vi "Dashboard Main.vi"() -> ()   [LabVIEW 2015]
uses:
  <vilib>/Utility/miscctls.llb/LVRowAndColumnTypeDef.ctl
  <vilib>/event_ctls.llb/eventvkey.ctl
  <vilib>/Rock Robotics/WPI/Dashboard/WPI_DashboardLogging Global.vi
  <vilib>/Rock Robotics/Network Tables/NT Read Boolean.vi
  <vilib>/Rock Robotics/Network Tables/NT Read Numeric Array.vi
  <vilib>/Utility/config.llb/Write Key (String).vi
  <vilib>/Utility/config.llb/Write Key (I32).vi
  <vilib>/Utility/config.llb/NI_LVConfig.lvlib
panel:
  in  "TCP":refnum<k5>
  in  "Rec Mode":enum32{"Stop", "Record", "Playback"}(radio)
  in  "Vision":u16(ring) items=["Camera Off", "USB Camera SW", "USB Camera HW", "IP Camera"]
  out "Camera IP":string
  out "Image Message":string="Timeout in Camera Communications"
  in  "Dashboard Tab":T1(tab)
  out "Joystick":dbl(knob) scale=0.0..360.0
  out "Encodeur 4":dbl
  out "Encodeur 3":dbl
  out "Encodeur 2":dbl
  out "encodeur 1":dbl
  in  "Select Auto":string(combo)
  out "NT Connection":bool
  in  "Camera Settings":T2={"Frame Rate"=30, "Compression"=30, "Size"=1} {"Frame Rate" scale=1.0..30.0; "Size" items=["640x480", "320x240", "160x120"]}
  out "MotorChart R":cluster{"Numeric":dbl, "Numeric":dbl}(graph)
  out "MotorChart L":T3(graph)
  out "MotorSliders R":cluster{"MotorSlide1":dbl, "MotorSlide2":dbl} {"MotorSlide2" scale=-1.0..1.0 scale format="%#_2e"; "MotorSlide1" scale=-1.0..1.0 scale format="%#_2e"}
  out "MotorSliders L":T4 {"MotorSlide4 2" scale=0.0..14.0 scale format="%#_2e"; "MotorSlide2" scale=-1.0..1.0 scale format="%#_2e"; "MotorSlide1" scale=-1.0..1.0 scale format="%#_2e"}
  out "orientation swerves":dbl(knob) scale=0.0..360.0
  out "JS1 Z":dbl(slide) scale=-1.0..1.0 scale format="%#_2e"
  out "JS1 Graph":cluster{"X":dbl, "Y":dbl}[](graph)
  out "JS1 Buttons":T5
  out "JS2 Z":dbl(slide) scale=-1.0..1.0 scale format="%#_2e"
  out "JS2 Graph":cluster{"X":dbl, "Y":dbl}[](graph)
  out "JS2 Buttons":T5
  out "Mode":T6(ring)=enum."Auto Disabled"
  in  "DB Camera Config":bool
  out "fps":dbl format="%#.1g"
  out "Mbps":dbl format="%#.1g"
  out "Mbps LED":bool
  in  "DB/String 9":string
  in  "DB/String 8":string
  in  "DB/String 7":string
  in  "DB/String 6":string
  in  "DB/String 5":string
  in  "DB/String 4":string
  in  "DB/String 3":string
  in  "DB/String 2":string
  in  "DB/String 1":string
  in  "DB/String 0":string
  in  "DB/Slider 0":dbl(slide) scale=0.0..5.0
  in  "DB/Slider 1":dbl(slide) scale=0.0..5.0
  in  "DB/Slider 2":dbl(slide) scale=0.0..5.0
  in  "DB/Slider 3":dbl(slide) scale=0.0..5.0
  out "DB/LED 3":bool
  out "DB/LED 2":bool
  out "DB/LED 1":bool
  out "DB/LED 0":bool
  in  "DB/Button 3":bool
  in  "DB/Button 2":bool
  in  "DB/Button 1":bool
  in  "DB/Button 0":bool caption="New Name"
  in  "Test Slider":dbl(slide) scale=0.0..100.0 scale format="%#_3g"
  in  "On/Off":bool caption="Solenoid"
  in  "Test Name":u16(ring) items=["Select the test to run..."]
  in  "Test Tree":string(tree)
  in  "Motor":cluster{"Value":dbl, "Enable":bool} {"Value" scale=-1.0..1.0 scale format="%#_3g"}
  out "Progress":T7 {"Test Progress" scale=0.0..100.0}
  in  "Rev/Fwd":cluster{"Forward":bool, "Reverse":bool}
  in  "Test Ring":u16(ring) items=["Monochrome", "Color"]
  out "Cmd Status":string
  in  "Execute Command":bool
  in  "Command Params":string[][](table)
  in  "Command Selection":i32(listbox)
  in  "CheckList":i32(listbox)
  out "Tree":string(tree)
  out "Camera Image":T8(plugin-control)
  out "Background":bool
  # "Left"
  # "Front"
  # "Right"
  # "Battery"
  # "This tab is a great place for autonomous settings and robot-specific values.\nPlace controls and indicators inside this tab and match name to\nDashboard Variables on robot. You can also delete this comment."
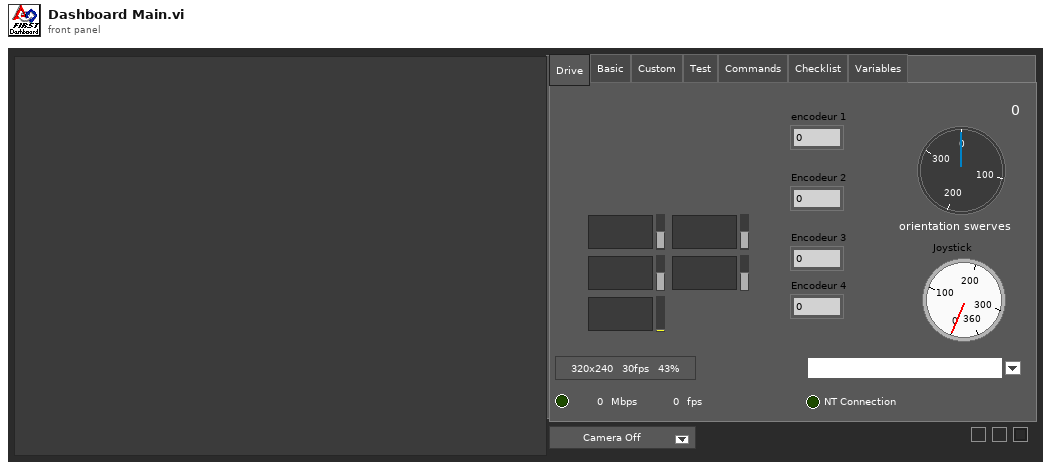
[diagram p1: front panel]
types:
  T1 = enum32{"Drive", "Basic", "Custom", "Test", "Commands", "Checklist", "Variables"}
  T2 = cluster{"Frame Rate":i32, "Compression":i32, "Size":u16}
  T3 = cluster{"Numeric":dbl, "Numeric":dbl, "Battery V":dbl}
  T4 = cluster{"MotorSlide1":dbl, "MotorSlide2":dbl, "MotorSlide4 2":dbl}
  T5 = cluster{bool, bool, bool, bool, bool, bool, bool, bool, bool, bool, bool, bool}
  T6 = enum8{"Tele-Op Disabled", "Tele-Op Enabled", "Auto Disabled", "Auto Enabled", "Test Disabled", "Test Enabled", "Disconnected", "No Code", "E-Stop"}
  T7 = cluster{"Test Progress":u8, "Test Progress Text":string}
  T8 = typedef "IMAQ Image.ctl" = refnum<image>
  T9 = cluster{"IDs":cluster{"RPC field ID":u16, "Unique ID":u16}, "String":string}
  T10 = enum32{"Drive", "Basic", "Custom", "Test", "Checklist", "Variables"}
  T11 = typedef "Image Type" = u32
  T12 = cluster{"Camera Image":refnum<vi>, "Dashboard Tab":refnum<vi>, "Background":refnum<vi>, "Vision":refnum<vi>, "Rec Mode":refnum<vi>, "Test Slider":refnum<vi>, "On/Off ":refnum<vi>, "Test Ring":refnum<vi>, "Rev/Fwd":refnum<vi>, "Test Name":refnum<vi>, "Motor":refnum<vi>, "Progress":refnum<vi>, "CheckList":refnum<vi>, "Tree":refnum<vi>, "Test Tree":refnum<vi>, "Command Params":refnum<vi>, "Command Selection":refnum<vi>, "Execute Command":refnum<vi>, "Cmd Status":refnum<vi>}
  T13 = cluster{"Error Strings":string, "Disable Counts":cluster{u16, u16}, "Rail Faults":cluster{u16, u16, u16}, "Robot IP":string, "DB Mode":u8, "Event Info":cluster{"Name":string, "Type":u8, "Number":u16, "Replay":u8}, "Camera Addr":string}
  T14 = cluster{"Storage":cluster{"Disk Free":u64, "RAM Block":u32, "RAM free":u32}, "CPU Utilization":cluster{"CPU % ISR":sgl, "CPU % Time Crit":sgl, "CPU % Timed Str":sgl, "CPU % High":sgl, "CPU % Above":sgl, "CPU % Normal":sgl, "CPU % Low":sgl}, "CAN":cluster{"% Bus Utilization":sgl, "Bus Off Cnt":u32, "TX_FIFO Full Cnt":u32, "Receive Error Cnt":u8, "Transmit Error Cnt":u8}, "HID":cluster{"HID Outputs":u32, "Rumble Low":u16, "Rumble High":u16}[]}
  T15 = cluster{"Status bits":cluster{"Test Mode":bool, "Autonomous":bool, "Enabled":bool, "Code Start":bool, "Brownout":bool, "Reserved 2":bool, "Reserved 3":bool, "E-Stop":bool}, "Code Trace":cluster{"Disabled":bool, "TeleOp":bool, "Auto":bool, "Test":bool}, "Controller Type":enum16{"unknown", "cRIO", "roboRio"}, "Code?":enum16{"unknown", "noCode", "code"}, "Battery V":dbl}
  T16 = cluster{"Control Bits":cluster{"TestMode":bool, "Autonomous":bool, "Enabled":bool, "FMS Present":bool, bool, bool, bool, "E-Stop":bool}, "Team Station ":u8, "Countdown":sgl, "Joystick Values":cluster{"Axes":dbl[], "Buttons":bool[], "POVs":i16[]}[]}
  T17 = cluster{"Axes":dbl[], "Buttons":bool[], "POVs":i16[]}[]
  T18 = cluster{"Axes":dbl[], "Buttons":bool[], "POVs":i16[]}
  T19 = cluster{"Buttons[0]":bool, "Buttons[1]":bool, "Buttons[2]":bool, "Buttons[3]":bool, "Buttons[4]":bool, "Buttons[5]":bool, "Buttons[6]":bool, "Buttons[7]":bool, "Buttons[8]":bool, "Buttons[9]":bool, "Buttons[10]":bool, "Buttons[11]":bool}
  T20 = typedef "NI_LVConfig.lvlib/Config Data RefNum.ctl" = refnum<k1>
  T21 = cluster{"Operation":enum16{"Update", "Clear"}, "Color Box":u32}[]
  T22 = typedef "eventvkey.ctl" = enum16{"ASCII", "Enter", "Return", "Shift", "Ctrl", "Alt", "Cmd", "Opt", "Caps", "NumLock", "Clear", "Break", "Up", "Down", "Left", "Right", "Insert", "Delete", "Home", "End", "PageUp", "PageDown", "Escape", "Help", "Pause", "ScrollLock", "F1", "F2", "F3", "F4", "F5", "F6", "F7", "F8", "F9", "F10", "F11", "F12", "F13", "F14", "F15", "F16", "F17", "F18", "F19", "F20", "F21", "F22", "F23", "F24", "Play", "VolumeUp", "VolumeDown", "Mute", "Two Byte Char"}
  T23 = cluster{"Image Size":bool, "Image Type":bool, "Pixel Value":bool, "ROI Information":bool, "Zoom Factor":bool}
  T24 = enum8{"Enabled", "Disabled", "Disabled and Grayed Out"}
  T25 = cluster{"Operation":enum16{"Update", "Clear"}, "Color Box":u32}
  T26 = typedef "LVRowAndColumnTypeDef.ctl" = cluster{"Row":i32, "Column":i32}
  T27 = cluster{"Shift":bool, "Ctrl":bool, "Alt":bool, "Cmd":bool, "Opt":bool}
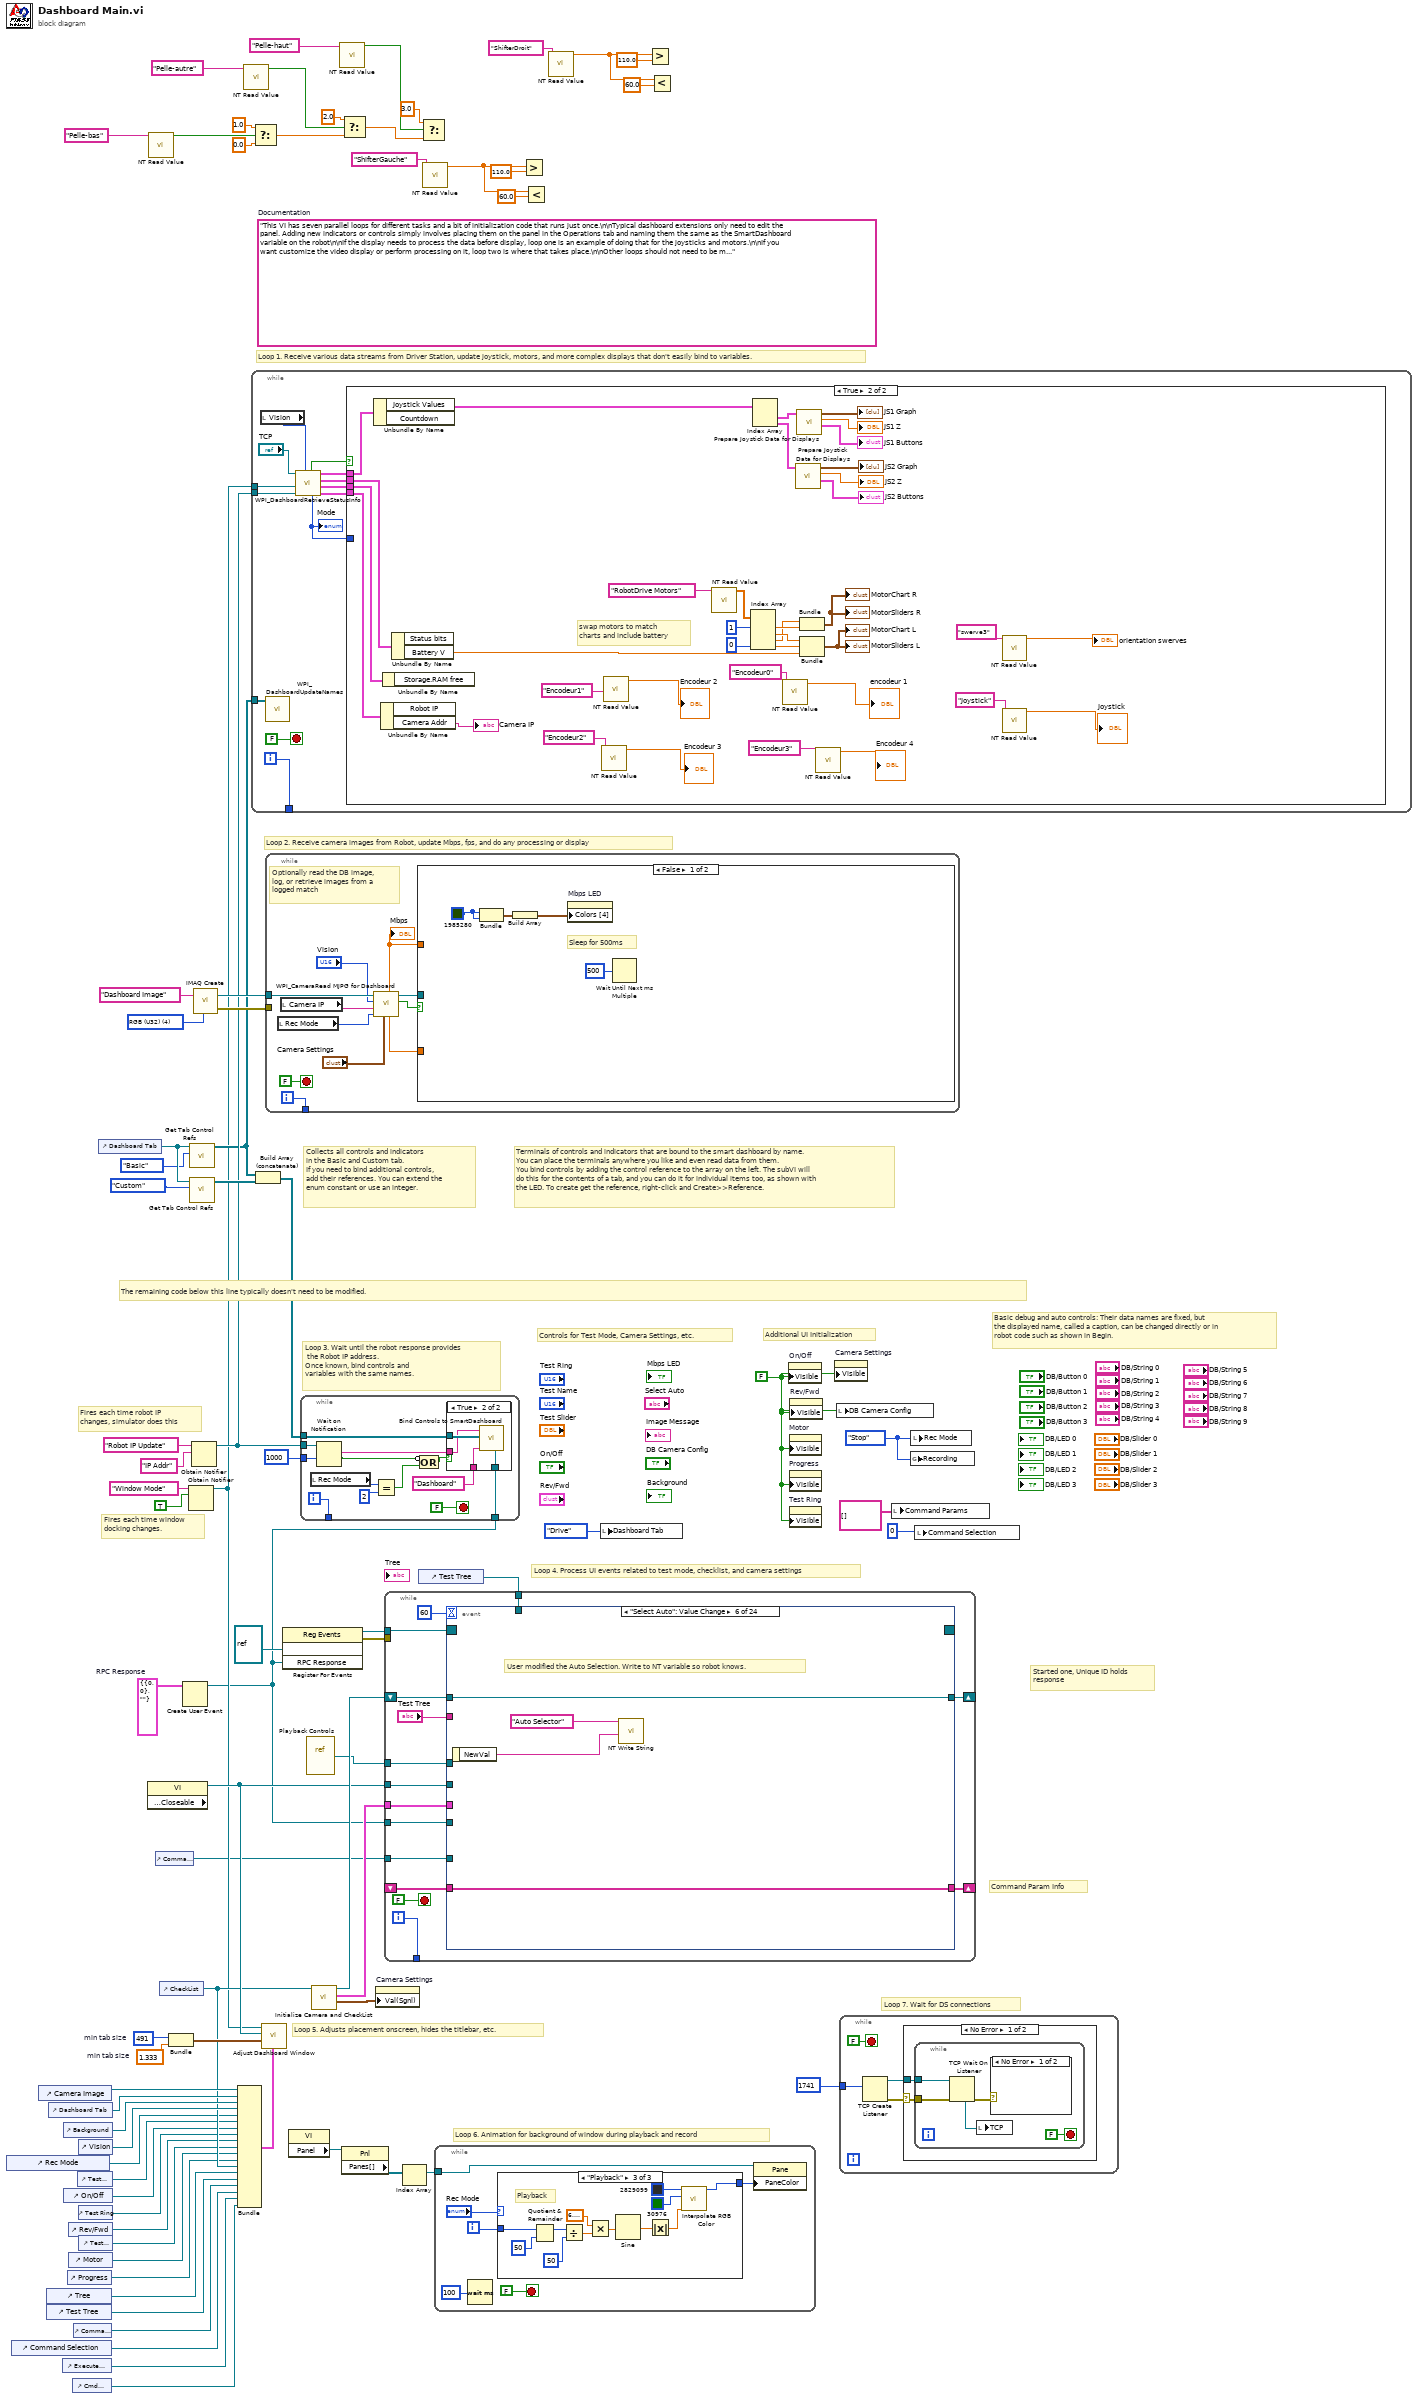
[diagram p0: block diagram]
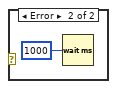
[diagram p2: hidden frame]
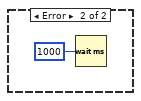
[diagram p3: hidden frame]
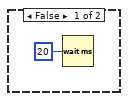
[diagram p4: hidden frame]
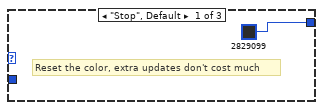
[diagram p5: hidden frame]
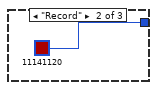
[diagram p6: hidden frame]
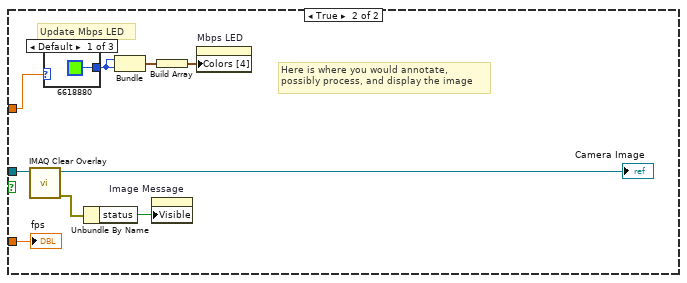
[diagram p8: hidden frame]
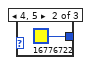
[diagram p9: hidden frame]
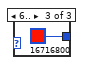
[diagram p10: hidden frame]
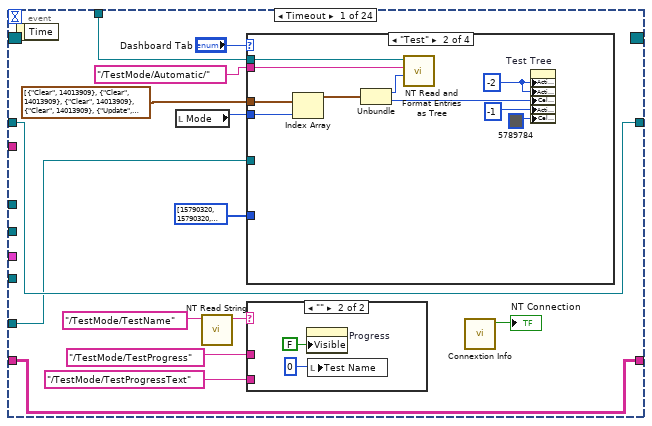
[diagram p11: hidden frame]
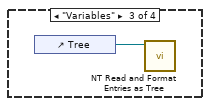
[diagram p13: hidden frame]
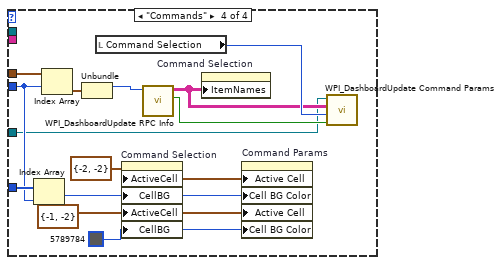
[diagram p14: hidden frame]
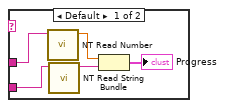
[diagram p15: hidden frame]
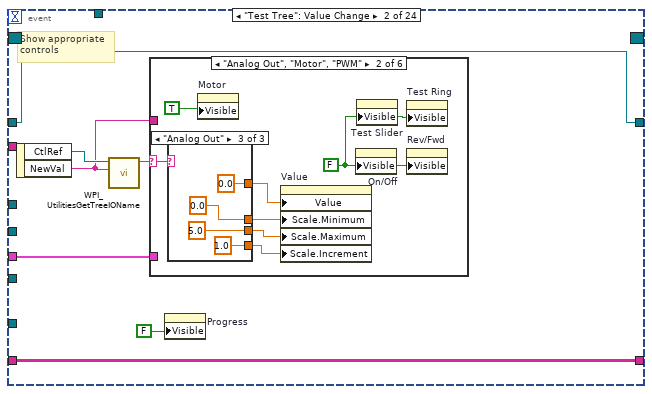
[diagram p16: hidden frame]
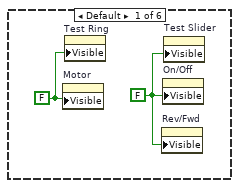
[diagram p17: hidden frame]
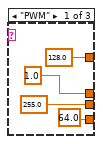
[diagram p18: hidden frame]
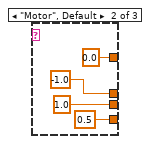
[diagram p19: hidden frame]
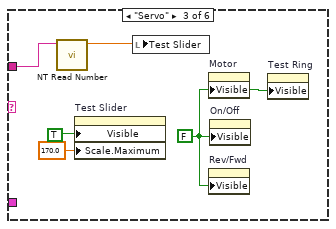
[diagram p20: hidden frame]
diagram:
  w27 = T9 {"IDs"={"RPC field ID"=0, "Unique ID"=0}, "String"=""}  # RPC Response
  w53 = 491  # min tab size
  w52 = 1.333  # min tab size
  w61 = enum32{"Stop", "Record", "Playback"}."Stop" ("Rec Mode")
  w35 = FALSE ("Visible")
  (unwired) "This VI has seven parallel loops for different tasks and a bit of initialization code that runs just once.\n\nTypical dashboard extensions only need to edit the panel. Adding new indicators or controls simply involves placing them on the panel in the Operations tab and naming them the same as the SmartDashboard variable on the robot\n\nIf the display needs to process the data before display, loop one is an example of doing that for the joysticks and motors.\n\nIf you want customize the video display or perform processing on it, loop two is where that takes place.\n\nOther loops should not need to be modified. They are pretty standard, and document the task they perform."  # Documentation
  w81 = T11 4 items=["Grayscale (U8)", "Grayscale (I16)", "Grayscale (SGL)", "Complex (CSG)", "RGB (U32)", "HSL (U32)", "RGB (U64)"] ("Image Type")
  # "Command Param Info"
  # "Started one, Unique ID holds\nresponse"
  # "Loop 7. Wait for DS connections"
  # "Basic debug and auto controls: Their data names are fixed, but\nthe displayed name, called a caption, can be changed directly or in\nrobot code such as shown in Begin."
  # "Controls for Test Mode, Camera Settings, etc."
  # "Additional UI Initialization"
  # "Loop 6. Animation for background of window during playback and record"
  # "Fires each time robot IP\nchanges, simulator does this"
  # "Fires each time window\ndocking changes."
  # "Collects all controls and indicators\nin the Basic and Custom tab.\nIf you need to bind additional controls,\nadd their references. You can extend the\nenum constant or use an integer."
  # "The remaining code below this line typically doesn't need to be modified."
  # "Loop 4. Process UI events related to test mode, checklist, and camera settings"
  # "Terminals of controls and indicators that are bound to the smart dashboard by name.\nYou can place the terminals anywhere you like and even read data from them.\nYou bind controls by adding the control reference to the array on the left. The subVI will\ndo this for the contents of a tab, and you can do it for individual items too, as shown with\nthe LED. To create get the reference, right-click and Create>>Reference."
  # "Loop 3. Wait until the robot response provides\n the Robot IP address.\nOnce known, bind controls and\nvariables with the same names."
  # "Loop 5. Adjusts placement onscreen, hides the titlebar, etc."
  # "Loop 1. Receive various data streams from Driver Station, update joystick, motors, and more complex displays that don't easily bind to variables."
  # "Loop 2. Receive camera images from Robot, update Mbps, fps, and do any processing or display"
  n1 = control-ref of="Rec Mode"() -> (w41:refnum<vi>)
  n2 = control-ref of="Command Selection"() -> (w26:refnum<vi>)
  n3 = control-ref of="Camera Image"() -> (w56:refnum<vi>)
  n4 = control-ref of="Tree"() -> (w45:refnum<vi>)
  n5 = control-ref of="Test Tree"() -> (w44:refnum<vi>)
  n6 = control-ref of="Dashboard Tab"() -> (w55:refnum<vi>)
  n7 = control-ref of="Execute Command"() -> (w28:refnum<vi>)
  n8 = control-ref of="Background"() -> (w50:refnum<vi>)
  n9 = control-ref of="On/Off"() -> (w39:refnum<vi>)
  n10 = control-ref of="Progress"() -> (w36:refnum<vi>)
  n11 = control-ref of="Rev/Fwd"() -> (w37:refnum<vi>)
  n12 = control-ref of="Motor"() -> (w42:refnum<vi>)
  n13 = control-ref of="Cmd Status"() -> (w22:refnum<vi>)
  n14 = control-ref of="Command Params"() -> (w29:refnum<vi>)
  n15 = control-ref of="Test Slider"() -> (w40:refnum<vi>)
  n16 = control-ref of="Vision"() -> (w54:refnum<vi>)
  n17 = control-ref of="Test Ring"() -> (w38:refnum<vi>)
  n18 = control-ref of="Test Name"() -> (w43:refnum<vi>)
  n19 = control-ref of="Dashboard Tab"() -> (w59:refnum<vi>)
  n20 = property class="VI" props=["Front Panel.Closeable"]() -> (reference out=w60:refnum<vi>)  [unwired: 2 in, 2 out]
  n21 = call-poly <vilib>:"NT Read Value.vi"("Name"="Pelle-bas") -> ("Boolean"=w14:bool)  [unwired: 9 in, 1 out]
  n22 = control-ref of="Command Params"() -> (w21:refnum<vi>)
  n23 = control-ref of="CheckList"() -> (w46:refnum<vi>)
  n24 = Bundle("min tab size"=w53, "min tab size"=w52) -> (w51:cluster{"min tab size":i32, "min tab size":dbl})  [unwired: 1 in]
  n25 = Create User Event(user event datatype=w27) -> (user event=w23:refnum<user-event>)  [unwired: 1 in, 1 out]
  n26 = Obtain Notifier(name (unnamed)="Window Mode", notification data type=TRUE) -> (notifier out=w32:refnum<notifier>)  [unwired: 2 in, 2 out]
  n27 = call <vilib>:"Get Tab Control Refs.vi"("Page Index"=T10."Basic" ("Dashboard Tab"), "TabControl in"=w59) -> ("ControlsOnPage"=w33:refnum<vi>[])  [unwired: 9 in]
  n28 = call <vilib>:"Get Tab Control Refs.vi"("Page Index"=T10."Custom" ("Dashboard Tab"), "TabControl in"=w59) -> ("ControlsOnPage"=w58:refnum<vi>[])  [unwired: 9 in]
  n29 = Obtain Notifier(name (unnamed)="Robot IP Update", notification data type="IP Addr" ("name (unnamed)")) -> (notifier out=w34:refnum<notifier>)  [unwired: 2 in, 2 out]
  n30 = call "IMAQ Create"("Image Name"="Dashboard Image", "Image Type"=w81) -> ("New Image"=w79:T8, "error out"=w78:errorcluster)  [unwired: 2 in, 1 out]
  n31 = Bundle("Camera Image"=w56, "Dashboard Tab"=w55, "Background"=w50, "Vision"=w54, "Rec Mode"=w41, "Test Slider"=w40, "On/Off"=w39, "Test Ring"=w38, "Rev/Fwd"=w37, "Test Name"=w43, "Motor"=w42, "Progress"=w36, "CheckList"=w46, "Tree"=w45, "Test Tree"=w44, "Command Params"=w29, "Command Selection"=w26, "Execute Command"=w28, "Cmd Status"=w22) -> (w47:T12)  [unwired: 1 in]
  n32 = call-poly <vilib>:"NT Read Value.vi"("Name"="Pelle-autre") -> ("Boolean"=w12:bool)  [unwired: 9 in, 1 out]
  n33 = while {
    tunnel: [w93] -> _
    tunnel: w34 -> [w87]
    tunnel: w33 -> [w86]
    tunnel: w32 -> [w82]
    i -> [w93]
    stop <- FALSE stop-if-true
    n34 = local read "Vision"() -> (w84:u16)
    n35 = call <vilib>:"WPI_DashboardUpdateNames.vi"("Controls on Tab"=w86) -> ()  [unwired: 11 in]
    n36 = call <vilib>:"WPI_DashboardRetrieveStatusInfo.vi"("Vision"=w84, "Binding Refnum"=w87, "Window Mode Notifier"=w82, "TCP Cnx"="TCP") -> ("Power and Errors"=w88:T13, "Robot Metrics"=w91:T14, "Status Info"=w92:T15, "Control Info"=w89:T16, "Robot Mode"=w85:T6, "Process?"=w90:bool)  [unwired: 2 in]
    "Mode" <- w85
    n37 = case shown="True" w90 {
      tunnel: w92 -> [_ w132]
      tunnel: w91 -> [_ w131]
      tunnel: w89 -> [_ w130]
      tunnel: w88 -> [_ w129]
      tunnel: w85 -> [_ _]
      frame False {
        n38 = Wait (ms)(milliseconds to wait=u32 20) -> ()  [unwired: 1 out]
      }
      frame True {
        # "swap motors to match\ncharts and include battery"
        n39 = Unbundle By Name(w130) -> ("Joystick Values"=w119:T17)  [unwired: 1 out]
        n40 = Unbundle By Name(w129) -> ("Camera Addr"=→"Camera IP":string)  [unwired: 1 out]
        n41 = Unbundle By Name(w131) -> ()  [unwired: 1 out]
        n42 = Unbundle By Name(w132) -> ("Battery V"=w120:dbl)  [unwired: 1 out]
        n43 = call-poly <vilib>:"NT Read Value.vi"("Name"="Encodeur2") -> ("Numeric"=→"Encodeur 3":dbl)  [unwired: 9 in, 1 out]
        n44 = call-poly <vilib>:"NT Read Value.vi"("Name"="Encodeur1") -> ("Numeric"=→"Encodeur 2":dbl)  [unwired: 9 in, 1 out]
        n45 = call-poly <vilib>:"NT Read Value.vi"("Name"="RobotDrive Motors") -> ("Numeric Array"=w108:dbl[])  [unwired: 9 in, 1 out]
        n46 = Index Array(array=w108, index #1=1, index #4=0) -> (element #1=w124:dbl, element #2=w125:dbl, element #3=w123:dbl, element #4=w128:dbl)  [unwired: 2 in]
        n47 = Index Array(array=w119) -> (element #1=w118:T18, element #2=w113:T18)  [unwired: 2 in]
        n48 = call-poly <vilib>:"NT Read Value.vi"("Name"="Encodeur0") -> ("Numeric"=→"encodeur 1":dbl)  [unwired: 9 in, 1 out]
        n49 = call "Prepare Joystick Data for Displays.vi"("Joystick Values"=w113) -> ("Buttons"=→"JS2 Buttons":T19, "Z Axis"=→"JS2 Z":dbl, "Cartesian Data"=→"JS2 Graph":cluster{"X axis":dbl, "X axis":dbl}[])  [unwired: 8 in]
        n50 = call "Prepare Joystick Data for Displays.vi"("Joystick Values"=w118) -> ("Buttons"=→"JS1 Buttons":T19, "Z Axis"=→"JS1 Z":dbl, "Cartesian Data"=→"JS1 Graph":cluster{"X axis":dbl, "X axis":dbl}[])  [unwired: 8 in]
        n51 = Bundle("Numeric"=w123, "Numeric"=w124) -> (→"MotorChart R" →"MotorSliders R":cluster{"Numeric":dbl, "Numeric":dbl})  [unwired: 1 in]
        n52 = Bundle("Numeric"=w125, "Numeric"=w128, "Battery V"=w120) -> (→"MotorChart L" →"MotorSliders L":T3)  [unwired: 1 in]
        n53 = call-poly <vilib>:"NT Read Value.vi"("Name"="Encodeur3") -> ("Numeric"=→"Encodeur 4":dbl)  [unwired: 9 in, 1 out]
        n54 = call-poly <vilib>:"NT Read Value.vi"("Name"="swerve3") -> ("Numeric"=→"orientation swerves":dbl)  [unwired: 9 in, 1 out]
        n55 = call-poly <vilib>:"NT Read Value.vi"("Name"="Joystick") -> ("Numeric"=→"Joystick":dbl)  [unwired: 9 in, 1 out]
      }
    }
  }
  n56 = Select(t=1.0, s=w14, f=0.0) -> (s? t:f=w11:dbl)
  n57 = Build Array (concatenate)(w33, w58) -> (w57:refnum<vi>[])
  n58 = call "Adjust Dashboard Window.vi"("Sizing Refnums"=w47, "Size Constraints"=w51, "VI"=w60, "WIn Mode"=w32) -> ()  [unwired: 8 in]
  n59 = while {
    tunnel: w79 -> [w141]
    tunnel: w78 -> [_]
    tunnel: [w142] -> _
    i -> [w142]
    stop <- FALSE stop-if-true
    # "Optionally read the DB image,\nlog, or retrieve images from a\nlogged match"
    n60 = local read "Rec Mode"() -> (w136:enum32{"Stop", "Record", "Playback"})
    n61 = local read "Camera IP"() -> (w134:string)
    n62 = call <vilib>:"WPI_CameraRead MJPG for Dashboard.vi"("Camera Settings"="Camera Settings", "Rec Mode"=w136, "Camera IP"=w134, "Camera Mode"="Vision", "Refnum in"=w141) -> ("Active"=w139:bool, "Refnum out"=w140:T8, "FPS"=w138:dbl, "Bandwidth (Mbps)"=w133:dbl)  [unwired: 3 in]
    "Mbps" <- w133
    n63 = case shown="False" w139 {
      tunnel: w140 -> [_ w151]
      tunnel: w133 -> [_ w150]
      tunnel: w138 -> [_ w148]
      frame False {
        w144 = u32 1985280 ("Color Box")
        # "Sleep for 500ms"
        n64 = Bundle("Color Box"=w144, "Color Box"=w144) -> (w146:cluster{"Color Box":u32, "Color Box":u32})  [unwired: 1 out]
        n65 = Build Array(w146) -> (w145:cluster{"Color Box":u32, "Color Box":u32}[])
        n66 = property on="Mbps LED" class="Bool (strict)"("Colors [4]"=w145) -> ()  [unwired: 2 in, 2 out]
        n67 = Wait Until Next ms Multiple(millisecond multiple=u32 500) -> ()  [unwired: 1 out]
      }
      frame True {
        # "Here is where you would annotate,\npossibly process, and display the image"
        # "Update Mbps LED"
        n68 = call "IMAQ Clear Overlay"("Image"=w151) -> ("error out"=w155:errorcluster, "Image Out"=→"Camera Image":T8)  [unwired: 2 in, 7 out]
        n69 = case shown="Default" w150 {
          tunnel: [u32 6618880 ("Color Box") u32 16776722 ("Color Box") u32 16716800 ("Color Box")] -> w152
          frame Default {
          }
          frame 4, 5 {
          }
          frame 6.. {
          }
        }
        n70 = Unbundle By Name(w155) -> ("status"=w156:bool)
        n71 = Bundle("Color Box"=w152, "Color Box"=w152) -> (w154:cluster{"Color Box":u32, "Color Box":u32})  [unwired: 1 out]
        n72 = property on="Image Message" class="Str"("Visible"=w156) -> ()  [unwired: 2 in, 2 out]
        n73 = Build Array(w154) -> (w153:cluster{"Color Box":u32, "Color Box":u32}[])
        n74 = property on="Mbps LED" class="Bool (strict)"("Colors [4]"=w153) -> ()  [unwired: 2 in, 2 out]
        "fps" <- w148
      }
    }
  }
  n75 = register-events(refnum<vi> refnum, w23) -> (reference out=w65:refnum<event-registration>, error out=w64:errorcluster)  [unwired: 2 in]
  n76 = property class="VI"() -> ("Panel"=w68:refnum<vi>)  [unwired: 2 in, 2 out]
  n77 = while {
    tunnel: w57 -> [w172]
    tunnel: w34 -> [w170]
    tunnel: [w168] -> _
    tunnel: u32 1000 ("milliseconds to wait") -> [w167]
    tunnel: w23 -> [w160]
    i -> [w168]
    stop <- FALSE stop-if-true
    n78 = local read "Rec Mode"() -> (w163:enum32{"Stop", "Record", "Playback"})
    n79 = Wait on Notification(notifier=w170, timeout in ms (-1)=w167) -> (notification=w169:string, timed out?=w165:bool)  [unwired: 2 in, 2 out]
    n80 = Equal?(x=w163, y=u16 2 ("Rec Mode")) -> (x = y?=w164:bool)
    n81 = Compound Arithmetic op=OR(invert w165, w164) -> (w166:bool)
    n82 = case shown="True" w166 {
      tunnel: w172 -> [_ w176]
      tunnel: w169 -> [_ w175]
      tunnel: "Dashboard" -> [_ w174]
      tunnel: w160 -> [_ w173]
      frame False {
      }
      frame True {
        n83 = call <vilib>:"Bind Controls to SmartDashboard.vi"("RPC ref"=w173, "Client Name"=w174, "Bound Control Refs"=w176, "Server IP Address"=w175) -> ()  [unwired: 8 in]
      }
    }
  }
  n84 = vi-ref "Playback Controls.vi"() -> (w66:refnum<vi>)
  n85 = call "Initialize Camera and CheckList.vi"("ListBox in"=w46) -> ("Cluster"=w72:cluster{"value":i32, "value":i32, "index":i32}, "Array"=w73:cluster{string[]}[], "File Refnum"=w71:T20)  [unwired: 8 in]
  n86 = call-poly <vilib>:"NT Read Value.vi"("Name"="Pelle-haut") -> ("Boolean"=w17:bool)  [unwired: 9 in, 1 out]
  n87 = property class="Pnl"(reference=w68) -> ("Panes[]"=w69:refnum<vi>[])  [unwired: 1 in, 2 out]
  n88 = Select(t=2.0, s=w12, f=w11) -> (s? t:f=w9:dbl)
  n89 = property on="Camera Settings" class="Clust (strict)"("Val(Sgnl)"=w72) -> ()  [unwired: 2 in, 2 out]
  n90 = Index Array(array=w69) -> (element=w67:refnum<vi>)  [unwired: 1 in]
  n91 = control-ref of="Test Tree"() -> (w70:refnum<vi>)
  n92 = while {
    tunnel: w73 -> [w188]
    shift-right: [w187] -> _
    shift-left: w71 -> [w186]
    tunnel: [w185] -> _
    tunnel: w70 -> [w184]
    tunnel: w66 -> [w183]
    tunnel: w65 -> [w182]
    tunnel: w64 -> [_]
    tunnel: w60 -> [w181]
    tunnel: w23 -> [w180]
    tunnel: w21 -> [w179]
    shift-right: [w178] -> _
    shift-left: _ -> [w177]
    i -> [w185]
    stop <- FALSE stop-if-true
    n93 = event shown="[5] \"Select Auto\": Value Change" {
      selector: w182 -> [_ _ _ _ _ _ _ _ _ _ _ _ _ _ _ _ _ _ _ _ _ _ _ _]
      dyn-events: [_ _ _ _ _ _ _ _ _ _ _ _ _ _ _ _ _ _ w497 _ _ _ _ _] -> _
      timeout: u32 60 ("milliseconds to wait") -> [_ _ _ _ _ _ _ _ _ _ _ _ _ _ _ _ _ _ _ _ _ _ _ _]
      tunnel: w184 -> [w201 _ _ _ _ _ _ _ _ _ _ _ _ _ _ _ _ _ _ _ _ _ _ _]
      tunnel: "Test Tree" -> [_ _ _ _ _ _ _ _ _ _ _ _ _ w460 w469 w472 w477 w486 _ _ _ _ _ _]
      tunnel: w188 -> [_ w239 _ _ _ _ _ _ _ _ _ w422 w453 _ _ _ _ _ _ _ _ _ _ _]
      tunnel: [w198 w238 w342 w348 w358 w362 w368 w380 w388 w394 w407 w421 w446 w459 w467 w471 w476 w485 w499 w515 w517 w525 w536 w541] -> w187
      tunnel: w186 -> [w198 w238 w342 w348 w358 w362 w368 w380 w388 w394 w407 w420 w446 w459 w467 w471 w476 w485 w499 w515 w517 w525 w536 w541]
      tunnel: w183 -> [_ _ _ _ _ _ _ _ _ _ _ _ _ _ _ _ _ _ w500 _ w520 _ _ _]
      tunnel: w181 -> [_ _ _ _ _ _ _ _ _ _ _ _ _ _ _ _ _ _ w495 _ _ _ _ _]
      tunnel: w180 -> [_ _ _ _ _ _ _ _ _ _ _ _ _ _ _ _ _ _ w491 _ _ _ _ _]
      tunnel: w179 -> [w193 _ _ _ _ _ w366 _ _ _ _ _ _ _ _ _ _ _ _ _ _ _ _ _]
      tunnel: [w192 w237 w341 w347 w357 w363 w364 w374 w385 w393 w406 w419 w445 w458 w466 w470 w475 w484 w490 w513 w516 w521 w529 w542] -> w178
      tunnel: w177 -> [w192 w237 w341 w347 w357 w363 w364 _ _ w393 w406 w419 w445 w458 w466 w470 w475 w484 w490 w513 w516 w521 w529 w542]
      event Timeout {
        n94 = event-data() -> ()  [unwired: 1 in, 1 out]
        n95 = local read "Mode"() -> (w195:T6)
        n96 = call <vilib>:"NT Read String.vi"("Name"="/TestMode/TestName") -> ("String"=w204:string)  [unwired: 9 in, 1 out]
        n97 = case shown="\"Test\"" "Dashboard Tab" {
          tunnel: w201 -> [_ w215 _ _]
          tunnel: "/TestMode/Automatic/" ("Name Pattern") -> [_ w214 _ _]
          tunnel: T21 [{"Operation"=enum."Clear", "Color Box"=14013909}, {"Operation"=enum."Clear", "Color Box"=14013909}, {"Operation"=enum."Clear", "Color Box"=14013909}, {"Operation"=enum."Clear", "Color Box"=14013909}, {"Operation"=enum."Update", "Color Box"=14013909}, {"Operation"=enum."Update", "Color Box"=16777215}, {"Operation"=enum."Clear", "Color Box"=14013909}, {"Operation"=enum."Clear", "Color Box"=14013909}, {"Operation"=enum."Clear", "Color Box"=14013909}] -> [_ w207 _ w224]
          tunnel: w195 -> [_ w206 _ w223]
          tunnel: u32[] [15790320, 15790320, 15790320, 15790320, 16777215, 16777215, 15790320, 15790320, 15790320] -> [_ _ _ w229]
          tunnel: w193 -> [_ _ _ w217]
          frame "Custom", Default {
          }
          frame "Test" {
            w213 = -2 ("Active Item:Row Number")
            n98 = Index Array(array=w207, index=w206) -> (element=w208:T25)
            n99 = Unbundle(w208) -> ("Operation"=w209:enum16{"Update", "Clear"}, "Color Box"=w210:u32)
            n100 = call <vilib>:"NT Read and Format Entries as Tree.vi"("Operation"=w209, "Name Pattern"=w214, "Tree Refnum"=w215) -> ()  [unwired: 7 in, 2 out]
            n101 = property on="Test Tree" class="Tree (strict)"("Active Item Row Number"=w213, "ActiveColNum"=w213, "CellBG"=w210, "Active Item Row Number"=-1 ("Active Item:Row Number"), "CellBG"=u32 5789784 ("Color Box")) -> ()  [unwired: 2 in, 2 out]
          }
          frame "Variables" {
            n102 = control-ref of="Tree"() -> (w216:refnum<vi>)
            n103 = call <vilib>:"NT Read and Format Entries as Tree.vi"("Tree Refnum"=w216) -> ()  [unwired: 9 in, 2 out]
          }
          frame "Commands" {
            w225 = u32 5789784 ("Color Box")
            w226 = T26 {"Row"=-1, "Column"=-2} ("Active Cell:Active Cell")
            w228 = T26 {"Row"=-2, "Column"=-2} ("Active Cell:Active Cell")
            n104 = Index Array(array=w229, index=w223) -> (element=w227:u32)
            n105 = Index Array(array=w224, index=w223) -> (element=w222:T25)
            n106 = Unbundle(w222) -> ("Operation"=w221:enum16{"Update", "Clear"})  [unwired: 1 out]
            n107 = local read "Command Selection"() -> (w220:i32)
            n108 = property on="Command Selection" class="MCListbox (strict)"("ActiveCell"=w228, "CellBG"=w227, "ActiveCell"=w226, "CellBG"=w225) -> ()  [unwired: 2 in, 2 out]
            n109 = call <vilib>:"WPI_DashboardUpdate RPC Info.vi"("Operation"=w221) -> ("update"=w219:bool, "commands"=w218:string[][])  [unwired: 9 in]
            n110 = property on="Command Selection" class="MCListbox (strict)"("ItemNames"=w218) -> ()  [unwired: 2 in, 2 out]
            n111 = property on="Command Params" class="Tbl (strict)"("Active Cell"=w228, "Cell BG Color"=w227, "Active Cell"=w226, "Cell BG Color"=w225) -> ()  [unwired: 2 in, 2 out]
            n112 = call <vilib>:"WPI_DashboardUpdate Command Params.vi"("Update"=w219, "NewVal"=w220, "Commands"=w218, "Param Tbl"=w217) -> ()  [unwired: 7 in, 1 out]
          }
        }
        n113 = case shown="\"\"" w204 {
          tunnel: "/TestMode/TestProgress" ("Name") -> [w231 _]
          tunnel: "/TestMode/TestProgressText" ("Name") -> [w230 _]
          frame Default {
            n114 = call <vilib>:"NT Read Number.vi"("Name"=w231) -> ("Numeric"=w232:dbl)  [unwired: 9 in, 1 out]
            n115 = call <vilib>:"NT Read String.vi"("Name"=w230) -> ("String"=w233:string)  [unwired: 9 in, 1 out]
            n116 = Bundle("Numeric"=w232, "String"=w233) -> (→"Progress":cluster{"Numeric":dbl, "String":string})  [unwired: 1 in]
          }
          frame "" {
            n117 = property on="Progress" class="Clust (strict)"("Visible"=FALSE) -> ()  [unwired: 2 in, 2 out]
            n118 = local write "Test Name"(u16 0) -> ()
          }
        }
        n119 = call <vilib>:"Connextion Info.vi"() -> ("Connected"=→"NT Connection":bool)  [unwired: 10 in, 1 out]
      }
      event "Test Tree": Value Change {
        # "Show appropriate\ncontrols"
        n120 = event-data() -> ("CtlRef"=w242:refnum<vi>, "NewVal"=w240:string)  [unwired: 1 in]
        n121 = call <vilib>:"WPI_UtilitiesGetTreeIOName.vi"("NewVal"=w240, "TreeControl in"=w242) -> ("I/O Name"=w243:string)  [unwired: 9 in]
        n122 = case shown="\"Analog Out\", \"Motor\", \"PWM\"" w243 {
          selector: w243 -> [_ w250 _ w272 w281 _]
          tunnel: w240 -> [_ _ w269 w271 _ w288]
          tunnel: w239 -> [_ _ _ _ _ w287]
          frame Default {
            w245 = FALSE ("Visible")
            w244 = FALSE ("Visible")
            n123 = property on="Motor" class="Clust (strict)"("Visible"=w244) -> ()  [unwired: 2 in, 2 out]
            n124 = property on="Test Ring" class="Ring (strict)"("Visible"=w244) -> ()  [unwired: 2 in, 2 out]
            n125 = property on="Rev/Fwd" class="Clust (strict)"("Visible"=w245) -> ()  [unwired: 2 in, 2 out]
            n126 = property on="On/Off" class="Bool (strict)"("Visible"=w245) -> ()  [unwired: 2 in, 2 out]
            n127 = property on="Test Slider" class="Slide (strict)"("Visible"=w245) -> ()  [unwired: 2 in, 2 out]
          }
          frame "Analog Out", "Motor", "PWM" {
            w251 = FALSE ("Visible")
            n128 = case shown="\"Analog Out\"" w250 {
              tunnel: [1.0 ("Value") -1.0 ("Value") 0.0 ("Value")] -> w249
              tunnel: [255.0 ("Value") 1.0 ("Value") 5.0 ("Value")] -> w248
              tunnel: [128.0 ("Value") 0.0 ("Value") 0.0 ("Value")] -> w247
              tunnel: [64.0 ("Value") 0.5 ("Value") 1.0 ("Value")] -> w246
              frame "PWM" {
              }
              frame "Motor", Default {
              }
              frame "Analog Out" {
              }
            }
            n129 = property on="Motor" class="Clust (strict)"("Visible"=TRUE) -> ()  [unwired: 2 in, 2 out]
            n130 = property on="Value" class="Slide (strict)"("Value"=w247, "Scale.Minimum"=w249, "Scale.Maximum"=w248, "Scale.Increment"=w246) -> ()  [unwired: 2 in, 2 out]
            n131 = property on="On/Off" class="Bool (strict)"("Visible"=w251) -> ()  [unwired: 2 in, 2 out]
            n132 = property on="Test Slider" class="Slide (strict)"("Visible"=w251) -> ()  [unwired: 2 in, 2 out]
            n133 = property on="Test Ring" class="Ring (strict)"("Visible"=w251) -> ()  [unwired: 2 in, 2 out]
            n134 = property on="Rev/Fwd" class="Clust (strict)"("Visible"=w251) -> ()  [unwired: 2 in, 2 out]
          }
          frame "Servo" {
            w267 = FALSE ("Visible")
            n135 = call <vilib>:"NT Read Number.vi"("Name"=w269) -> ("Numeric"=w268:dbl)  [unwired: 9 in, 1 out]
            n136 = property on="Test Slider" class="Slide (strict)"("Visible"=TRUE, "Scale.Maximum"=170.0 ("Scale.Range:Maximum")) -> ()  [unwired: 2 in, 2 out]
            n137 = local write "Test Slider"(w268) -> ()
            n138 = property on="Motor" class="Clust (strict)"("Visible"=w267) -> ()  [unwired: 2 in, 2 out]
            n139 = property on="Rev/Fwd" class="Clust (strict)"("Visible"=w267) -> ()  [unwired: 2 in, 2 out]
            n140 = property on="On/Off" class="Bool (strict)"("Visible"=w267) -> ()  [unwired: 2 in, 2 out]
            n141 = property on="Test Ring" class="Ring (strict)"("Visible"=w267) -> ()  [unwired: 2 in, 2 out]
          }
          frame "Relay", "Solenoid" {
            w270 = FALSE ("Visible")
            n142 = property on="Motor" class="Clust (strict)"("Visible"=w270) -> ()  [unwired: 2 in, 2 out]
            n143 = property on="Test Slider" class="Slide (strict)"("Visible"=w270) -> ()  [unwired: 2 in, 2 out]
            n144 = Search and Replace String(input string=w271, search string="/Value  **", replace string="/Direction") -> (result string=w277:string)  [unwired: 5 in, 3 out]
            n145 = property on="Test Ring" class="Ring (strict)"("Visible"=w270) -> ()  [unwired: 2 in, 2 out]
            n146 = call <vilib>:"NT Read String.vi"("Name"=w277) -> ("String"=w275:string)  [unwired: 9 in, 1 out]
            n147 = Equal?(x="Both directions", y=w275) -> (x = y?=w273:bool)
            n148 = Not(x=w273) -> (.not. x?=w274:bool)
            n149 = property on="Rev/Fwd" class="Clust (strict)"("Visible"=w273) -> ()  [unwired: 2 in, 2 out]
            n150 = property on="On/Off" class="Bool (strict)"("Visible"=w274, "Caption.Text"=w272) -> ()  [unwired: 2 in, 2 out]
          }
          frame "Compressor", "Digital Out" {
            w280 = FALSE ("Visible")
            # "Get direction and finish"
            n151 = property on="Motor" class="Clust (strict)"("Visible"=w280) -> ()  [unwired: 2 in, 2 out]
            n152 = property on="Test Slider" class="Slide (strict)"("Visible"=w280) -> ()  [unwired: 2 in, 2 out]
            n153 = property on="Test Ring" class="Ring (strict)"("Visible"=w280) -> ()  [unwired: 2 in, 2 out]
            n154 = property on="On/Off" class="Bool (strict)"("Visible"=TRUE, "Caption.Text"=w281) -> ()  [unwired: 2 in, 2 out]
            n155 = property on="Rev/Fwd" class="Clust (strict)"("Visible"=FALSE) -> ()  [unwired: 2 in, 2 out]
          }
          frame "Camera" {
            n156 = call <vilib>:"Get Last Path Segment.vi"("String in"=w288) -> ("String out"=w289:string)  [unwired: 10 in]
            n157 = property on="On/Off" class="Bool (strict)"("Visible"=FALSE) -> ()  [unwired: 2 in, 2 out]
            n158 = property on="Motor" class="Clust (strict)"("Visible"=FALSE) -> ()  [unwired: 2 in, 2 out]
            n159 = property on="Rev/Fwd" class="Clust (strict)"("Visible"=FALSE) -> ()  [unwired: 2 in, 2 out]
            n160 = case shown="\"White Balance  **\"" w289 {
              tunnel: w288 -> [w295 w304 w313 w322 w331 _ w337]
              tunnel: w287 -> [w293 w301 w310 w319 w328 _ _]
              frame "Size  **" {
                n161 = Index Array(array=w293) -> (element=w292:cluster{string[]})  [unwired: 1 in]
                n162 = call <vilib>:"NT Read String.vi"("Name"=w295) -> ("String"=w294:string)  [unwired: 9 in, 1 out]
                n163 = Unbundle(w292) -> (w290:string[])
                n164 = Match First String(2:w290, 3:w294) -> (0:w291:i32)  [unwired: 1 out]
                n165 = property on="Test Ring" class="Ring (strict)"("Value"=w291, "Strings []"=w290) -> ()  [unwired: 2 in, 2 out]
                n166 = property on="Test Ring" class="Ring (strict)"("Visible"=TRUE) -> ()  [unwired: 2 in, 2 out]
                n167 = property on="Test Slider" class="Slide (strict)"("Visible"=FALSE) -> ()  [unwired: 2 in, 2 out]
              }
              frame "White Balance  **" {
                n168 = Index Array(array=w301, index=1) -> (element=w302:cluster{string[]})
                n169 = call <vilib>:"NT Read String.vi"("Name"=w304) -> ("String"=w303:string)  [unwired: 9 in, 1 out]
                n170 = Unbundle(w302) -> (w299:string[])
                n171 = Match First String(2:w299, 3:w303) -> (0:w298:i32)  [unwired: 1 out]
                n172 = property on="Test Ring" class="Ring (strict)"("Value"=w298, "Strings []"=w299) -> ()  [unwired: 2 in, 2 out]
                n173 = property on="Test Ring" class="Ring (strict)"("Visible"=TRUE) -> ()  [unwired: 2 in, 2 out]
                n174 = property on="Test Slider" class="Slide (strict)"("Visible"=FALSE) -> ()  [unwired: 2 in, 2 out]
              }
              frame "Exposure  **" {
                n175 = Index Array(array=w310, index=2) -> (element=w311:cluster{string[]})
                n176 = call <vilib>:"NT Read String.vi"("Name"=w313) -> ("String"=w312:string)  [unwired: 9 in, 1 out]
                n177 = Unbundle(w311) -> (w307:string[])
                n178 = Match First String(2:w307, 3:w312) -> (0:w308:i32)  [unwired: 1 out]
                n179 = property on="Test Ring" class="Ring (strict)"("Value"=w308, "Strings []"=w307) -> ()  [unwired: 2 in, 2 out]
                n180 = property on="Test Ring" class="Ring (strict)"("Visible"=TRUE) -> ()  [unwired: 2 in, 2 out]
                n181 = property on="Test Slider" class="Slide (strict)"("Visible"=FALSE) -> ()  [unwired: 2 in, 2 out]
              }
              frame "Exposure Priority  **" {
                n182 = Index Array(array=w319, index=3) -> (element=w320:cluster{string[]})
                n183 = call <vilib>:"NT Read String.vi"("Name"=w322) -> ("String"=w321:string)  [unwired: 9 in, 1 out]
                n184 = Unbundle(w320) -> (w316:string[])
                n185 = Match First String(2:w316, 3:w321) -> (0:w317:i32)  [unwired: 1 out]
                n186 = property on="Test Ring" class="Ring (strict)"("Value"=w317, "Strings []"=w316) -> ()  [unwired: 2 in, 2 out]
                n187 = property on="Test Ring" class="Ring (strict)"("Visible"=TRUE) -> ()  [unwired: 2 in, 2 out]
                n188 = property on="Test Slider" class="Slide (strict)"("Visible"=FALSE) -> ()  [unwired: 2 in, 2 out]
              }
              frame "Color Enable  **" {
                n189 = Index Array(array=w328, index=4) -> (element=w329:cluster{string[]})
                n190 = call <vilib>:"NT Read String.vi"("Name"=w331) -> ("String"=w330:string)  [unwired: 9 in, 1 out]
                n191 = Unbundle(w329) -> (w325:string[])
                n192 = Match First String(2:w325, 3:w330) -> (0:w326:i32)  [unwired: 1 out]
                n193 = property on="Test Ring" class="Ring (strict)"("Value"=w326, "Strings []"=w325) -> ()  [unwired: 2 in, 2 out]
                n194 = property on="Test Ring" class="Ring (strict)"("Visible"=TRUE) -> ()  [unwired: 2 in, 2 out]
                n195 = property on="Test Slider" class="Slide (strict)"("Visible"=FALSE) -> ()  [unwired: 2 in, 2 out]
              }
              frame Default {
                n196 = property on="Test Ring" class="Ring (strict)"("Visible"=FALSE) -> ()  [unwired: 2 in, 2 out]
                n197 = property on="Test Slider" class="Slide (strict)"("Visible"=FALSE) -> ()  [unwired: 2 in, 2 out]
              }
              frame "Brightness  **", "Color Level  **", "Compression  **", "FPS  **", "Sharpness  **" {
                n198 = call <vilib>:"NT Read Number.vi"("Name"=w337) -> ("Numeric"=w336:dbl)  [unwired: 9 in, 1 out]
                n199 = local write "Test Slider"(w336) -> ()
                n200 = property on="Test Slider" class="Slide (strict)"("Visible"=TRUE, "Scale.Maximum"=100.0 ("Scale.Range:Maximum")) -> ()  [unwired: 2 in, 2 out]
                n201 = property on="Test Ring" class="Ring (strict)"("Visible"=FALSE) -> ()  [unwired: 2 in, 2 out]
              }
            }
          }
        }
        n202 = property on="Progress" class="Clust (strict)"("Visible"=FALSE) -> ()  [unwired: 2 in, 2 out]
      }
      event "Test Name": Mouse Enter {
        # "Populate the ring with the list of tests"
        n203 = event-data() -> ()  [unwired: 1 in, 1 out]
        n204 = call <vilib>:"NT Read String Array.vi"("Name"="/TestMode/TestList") -> ("String Array"=w346:string[])  [unwired: 9 in, 1 out]
        n205 = Build Array (concatenate)("Select the test to run...", w346) -> (w345:string[])
        n206 = property on="Test Name" class="Ring (strict)"("Strings []"=w345) -> ()  [unwired: 2 in, 2 out]
      }
      event "Test Name": Value Change {
        w349 = FALSE ("Visible")
        # "Tell the robot the test name to run"
        n207 = event-data() -> ("NewVal"=w353:u16)  [unwired: 1 in]
        n208 = property on="Test Name" class="Ring (strict)"() -> ("Strings []"=w354:string[])  [unwired: 2 in, 2 out]
        n209 = local write "Progress"(T7 {"Test Progress"=0, "Test Progress Text"=""} ("Progress")) -> ()
        n210 = Index Array(array=w354, index=w353) -> (element=w352:string)
        n211 = call <vilib>:"NT Write String.vi"("String"=w352, "Name"="/TestMode/TestName") -> ()  [unwired: 9 in, 1 out]
        n212 = property on="Progress" class="Clust (strict)"("Visible"=TRUE) -> ()  [unwired: 2 in, 2 out]
        n213 = property on="Motor" class="Clust (strict)"("Visible"=w349) -> ()  [unwired: 2 in, 2 out]
        n214 = property on="Test Slider" class="Slide (strict)"("Visible"=w349) -> ()  [unwired: 2 in, 2 out]
        n215 = property on="On/Off" class="Bool (strict)"("Visible"=w349) -> ()  [unwired: 2 in, 2 out]
        n216 = property on="Rev/Fwd" class="Clust (strict)"("Visible"=w349) -> ()  [unwired: 2 in, 2 out]
        n217 = property on="Test Ring" class="Ring (strict)"("Visible"=w349) -> ()  [unwired: 2 in, 2 out]
      }
      event "Select Auto": Mouse Enter {
        # "Populate the combo box with the list of autonomous options"
        n218 = event-data() -> ()  [unwired: 1 in, 1 out]
        n219 = call <vilib>:"NT Read String Array.vi"("Name"="Auto List") -> ("String Array"=w356:string[])  [unwired: 9 in, 1 out]
        n220 = property on="Select Auto" class="CmbBox"("Strings[]"=w356) -> ()  [unwired: 2 in, 2 out]
      }
      event "Select Auto": Value Change {
        # "User modified the Auto Selection. Write to NT variable so robot knows."
        n221 = event-data() -> ("NewVal"=w360:string)  [unwired: 1 in]
        n222 = call <vilib>:"NT Write String.vi"("String"=w360, "Name"="Auto Selector") -> ()  [unwired: 9 in, 1 out]
      }
      event "Command Selection": Value Change {
        # "Get the params and show in table"
        n223 = event-data() -> ("NewVal"=w367:i32)  [unwired: 1 in]
        n224 = property on="Command Selection" class="MCListbox (strict)"() -> ("ItemNames"=w365:string[][])  [unwired: 2 in, 2 out]
        n225 = call <vilib>:"WPI_DashboardUpdate Command Params.vi"("NewVal"=w367, "Commands"=w365, "Param Tbl"=w366) -> ()  [unwired: 8 in, 1 out]
      }
      event "Execute Command": Value Change {
        # "Started one, Unique ID holds\nresponse"
        n226 = event-data() -> ()  [unwired: 1 in, 1 out]
        n227 = property on="Command Selection" class="MCListbox (strict)"() -> ("ItemNames"=w379:string[][])  [unwired: 2 in, 2 out]
        n228 = Index Array(array=w379, index (row)="Command Selection", index (col)=0) -> (element=w377:string)
        n229 = call <vilib>:"Invoke Commands.vi"("Command Params"="Command Params", "Function Name"=w377) -> ("Params"=w373:u8, "Started"=w372:bool)  [unwired: 7 in, 1 out]
        n230 = Array Subset(array="Command Params", length (row)=w373) -> (w374:string[][])  [unwired: 3 in]
        n231 = Select(t="Executing" ("Cmd Status"), s=w372, f="" ("Cmd Status")) -> (s? t:f=→"Cmd Status":string)
      }
      event "Command Selection": Double Click {
        n232 = event-data() -> ("Row"=w389:i32)  [unwired: 1 in]
        n233 = property on="Command Selection" class="MCListbox (strict)"() -> ("ItemNames"=w392:string[][])  [unwired: 2 in, 2 out]
        n234 = local read "Command Params"() -> (w387:string[][])
        n235 = Index Array(array=w392, index (row)=w389, index (col)=0) -> (element=w390:string)
        n236 = call <vilib>:"Invoke Commands.vi"("Command Params"=w387, "Function Name"=w390) -> ("Params"=w386:u8, "Started"=w381:bool)  [unwired: 7 in, 1 out]
        n237 = Array Subset(array=w387, length (row)=w386) -> (w385:string[][])  [unwired: 3 in]
        n238 = Select(t="Executing" ("Cmd Status"), s=w381, f="" ("Cmd Status")) -> (s? t:f=w382:string)
        n239 = local write "Cmd Status"(w382) -> ()
      }
      event "CheckList": Double Click {
        # "Shift clears all"
        # "Update symbols on the listbox"
        n240 = event-data() -> ("PlatMods.Shift"=w395:bool, "Row"=w397:i32)  [unwired: 1 in]
        n241 = case shown="True" w395 {
          tunnel: w397 -> [w401 _]
          tunnel: 1 -> [w400 _]
          frame False {
            n242 = property on="CheckList" class="LstBox (strict)"() -> ("Item Symbols"=w399:i32[])  [unwired: 2 in, 2 out]
            n243 = Replace Array Subset(array=w399, new element=w400, index=w401) -> (w398:i32[])
            n244 = property on="CheckList" class="LstBox (strict)"("Item Symbols"=w398) -> ()  [unwired: 2 in, 2 out]
          }
          frame True {
            w402 = 0 ("Top Row")
            n245 = property on="CheckList" class="LstBox (strict)"() -> ("Number of Rows"=w404:u32)  [unwired: 2 in, 2 out]
            n246 = Initialize Array(0, w404) -> (w403:i32[])
            n247 = property on="CheckList" class="LstBox (strict)"("Top Row"=w402, "Value"=w402, "Item Symbols"=w403) -> ()  [unwired: 2 in, 2 out]
          }
        }
      }
      event "CheckList": Key Down {
        # "Update symbols on the listbox\nLeft and right keys check and uncheck"
        n248 = event-data() -> ("VKey"=w409:T22)  [unwired: 1 in]
        n249 = case shown="\"Left\", \"Right\"" w409 {
          selector: w409 -> [w414 _]
          tunnel: eventvkey."Left" ("VKey") -> [w412 _]
          frame "Left", "Right" {
            n250 = Equal?(x=w412, y=w414) -> (x = y?=w413:bool)
            n251 = Select(t=0, s=w413, f=1) -> (s? t:f=w415:i32)
            n252 = property on="CheckList" class="LstBox (strict)"() -> ("Item Symbols"=w418:i32[])  [unwired: 2 in, 2 out]
            n253 = Replace Array Subset(array=w418, new element=w415, index="CheckList") -> (w417:i32[])
            n254 = property on="CheckList" class="LstBox (strict)"("Item Symbols"=w417) -> ()  [unwired: 2 in, 2 out]
          }
          frame Default {
          }
        }
      }
      event "DB Camera Config": Value Change {
        # "Show or hide the cluster of controls, store in ini file"
        n255 = event-data() -> ("NewVal"=w423:bool)  [unwired: 1 in]
        n256 = case shown="False" w423 {
          tunnel: w422 -> [w432 _]
          tunnel: [w425 w443] -> w421
          tunnel: w420 -> [w424 w443]
          frame False {
            w439 = "Camera"
            w442 = FALSE ("Visible")
            n257 = local read "Camera Settings"() -> (w431:T2)
            n258 = Index Array(array=w432) -> (element=w435:cluster{string[]})  [unwired: 1 in]
            n259 = Unbundle(w431) -> ("Frame Rate"=w430:i32, "Compression"=w429:i32, "Size"=w433:u16)
            n260 = Unbundle(w435) -> (w434:string[])
            n261 = Index Array(array=w434, index=w433) -> (element=w428:string)
            n262 = call-poly <vilib>:"Write Key.vi"("section"=w439, "value"=w428, "key"="Size", "refnum"=w424) -> ("refnum out"=w441:T20)  [unwired: 2 in, 5 out]
            n263 = call-poly <vilib>:"Write Key.vi"("section"=w439, "value"=w430, "key"="FrameRate", "refnum"=w441) -> ("refnum out"=w440:T20)  [unwired: 1 in, 6 out]
            n264 = property on="Camera Settings" class="Clust (strict)"("Visible"=w442) -> ()  [unwired: 2 in, 2 out]
            n265 = local write "DB Camera Config"(w442) -> ()
            n266 = call-poly <vilib>:"Write Key.vi"("section"=w439, "value"=w429, "key"="Compression", "refnum"=w440) -> ("refnum out"=w426:T20)  [unwired: 1 in, 6 out]
            n267 = call <vilib>:"Close Config Data.vi"("refnum"=w426) -> ("file path"=w427:path)  [unwired: 2 in, 8 out]
            n268 = call <vilib>:"Open Config Data.vi"("configuration file path"=w427) -> ("refnum"=w425:T20)  [unwired: 8 in, 2 out]
          }
          frame True {
            n269 = property on="Camera Settings" class="Clust (strict)"("Visible"=TRUE) -> ()  [unwired: 2 in, 2 out]
          }
        }
      }
      event "Camera Settings": Value Change {
        # "Update summary string when any elements of DB camera change"
        n270 = event-data() -> ("NewVal"=w457:T2)  [unwired: 1 in]
        n271 = Index Array(array=w453) -> (element=w452:cluster{string[]})  [unwired: 1 in]
        n272 = Unbundle(w457) -> ("Frame Rate"=w448:i32, "Compression"=w447:i32, "Size"=w450:u16)
        n273 = Unbundle(w452) -> (w451:string[])
        n274 = Index Array(array=w451, index=w450) -> (element=w449:string)
        n275 = Format Into String(format string="%s   %dfps   %d%%", w449, w448, w447) -> (resulting string=w454:string)  [unwired: 2 in, 1 out]
        n276 = Build Array(w454) -> (w455:string[])
        n277 = property on="DB Camera Config" class="Bool (strict)"("Strings [4]"=w455) -> ()  [unwired: 2 in, 2 out]
      }
      event "Motor.Enable": Value Change {
        # "When the test mode otor enable helper is set, update that\ntree row item's value"
        n278 = event-data() -> ("NewVal"=w464:bool)  [unwired: 1 in]
        n279 = Unbundle("Motor") -> ("Value"=w463:dbl)  [unwired: 1 out]
        n280 = Select(t=w463, s=w464, f=0.0) -> (s? t:f=w461:dbl)
        n281 = call <vilib>:"NT Write Number.vi"("Numeric"=w461, "Name"=w460) -> ()  [unwired: 9 in, 1 out]
      }
      event "Test Slider": Value Change {
        # "When the test mode slider helper is set, update that\ntree row item's value"
        n282 = event-data() -> ("NewVal"=w468:dbl)  [unwired: 1 in]
        n283 = call <vilib>:"NT Write Number.vi"("Numeric"=w468, "Name"=w469) -> ()  [unwired: 9 in, 1 out]
      }
      event "On/Off": Value Change {
        # "When the test mode on/off helper value is set, update that\ntree row item's value"
        n284 = event-data() -> ("NewVal"=w474:bool)  [unwired: 1 in]
        n285 = Boolean To (0,1)(Boolean=w474) -> (0, 1=w473:i16)
        n286 = call <vilib>:"NT Write Number.vi"("Numeric"=w473, "Name"=w472) -> ()  [unwired: 9 in, 1 out]
      }
      event "Rev/Fwd": Value Change {
        # "When the test mode helper value for relays is set, update that\ntree row item's value"
        n287 = event-data() -> ("NewVal.Forward"=w483:bool, "NewVal.Reverse"=w482:bool)  [unwired: 1 in]
        n288 = Boolean To (0,1)(Boolean=w483) -> (0, 1=w479:i16)
        n289 = Boolean To (0,1)(Boolean=w482) -> (0, 1=w481:i16)
        n290 = Negate(x=w481) -> (-x=w480:i16)
        n291 = Add(x=w479, y=w480) -> (x+y=w478:i16)
        n292 = call <vilib>:"NT Write Number.vi"("Numeric"=w478, "Name"=w477) -> ()  [unwired: 9 in, 1 out]
      }
      event "Test Ring": Value Change {
        # "When a test mode helper value is selected from the ring,\nset the tree item's variable to the string value"
        n293 = event-data() -> ("NewVal"=w488:u16)  [unwired: 1 in]
        n294 = property on="Test Ring" class="Ring (strict)"() -> ("Strings []"=w489:string[])  [unwired: 2 in, 2 out]
        n295 = Index Array(array=w489, index=w488) -> (element=w487:string)
        n296 = call <vilib>:"NT Write String.vi"("String"=w487, "Name"=w486) -> ()  [unwired: 9 in, 1 out]
      }
      event "Rec Mode": Value Change {
        # "Update globals for recording mode and path to read log from.\nClear when logging and let NetworkTables set path for vision to\nuse."
        n297 = event-data() -> ("NewVal"=w501:enum32{"Stop", "Record", "Playback"})  [unwired: 1 in]
        n298 = global write "WPI_DashboardLogging Global.vi" "Logging Filename"(path "") -> ()
        n299 = global write "WPI_DashboardLogging Global.vi" "Recording"(w501) -> ()
        n300 = case shown="\"Playback\"" w501 {
          tunnel: w500 -> [_ w503 w512]
          tunnel: [_ _ w511] -> w497
          tunnel: [_ _ w510] -> _
          tunnel: w495 -> [_ _ w508]
          tunnel: cluster{i32, i32} {-250, 170} -> [_ _ w507]
          tunnel: [_ _ T23 {"Image Size"=TRUE, "Image Type"=TRUE, "Pixel Value"=TRUE, "ROI Information"=TRUE, "Zoom Factor"=FALSE} ("Image Information Shown:All Elements")] -> w493
          tunnel: [_ _ TRUE ("Zoom Factor")] -> w492
          tunnel: w491 -> [_ _ w504]
          frame Default {
          }
          frame "Stop", "Record" {
            # "Place Window too"
            n301 = invoke class="VI" method="FP.Close"(reference=w503) -> (reference out=w502:refnum<vi>)  [unwired: 2 in, 2 out]
            n302 = invoke class="VI" method="Abort VI"(reference=w502) -> ()  [unwired: 2 in, 3 out]
          }
          frame "Playback" {
            n303 = call "Open Playback Panel.vi"("Offset"=w507, "DB VI Ref"=w508, "Playback in"=w512) -> ("Playback out"=w509:refnum<vi>)  [unwired: 8 in]
            n304 = register-events(w509, w504) -> (reference out=w511:refnum<event-registration>, error out=w510:errorcluster)  [unwired: 2 in]
          }
        }
        n305 = property on="Camera Image" class="ImageControl"("Image Information Shown"=w493, "Image Information Visible"=w492) -> ()  [unwired: 2 in, 2 out]
        n306 = call <vilib>:"WPI_DashboardNT Log FieldName Cache.vi"("Operation"=enum16{"Lookup/Add", "Index", "Clear"}."Clear") -> ()  [unwired: 8 in, 3 out]
      }
      event Panel Close {
        w514 = enum32{"Stop", "Record", "Playback"}."Stop" ("Rec Mode")
        # "Playback window has been closed, abort"
        n307 = event-data() -> ()  [unwired: 1 in, 4 out]
        n308 = local write "Rec Mode"(w514) -> ()
        n309 = global write "WPI_DashboardLogging Global.vi" "Recording"(w514) -> ()
      }
      event Panel Close {
        # "Abort playback window and ourself"
        n310 = event-data() -> ()  [unwired: 1 in, 4 out]
        n311 = invoke class="VI" method="FP.Close"(reference=w520) -> (reference out=w519:refnum<vi>)  [unwired: 2 in, 2 out]
        n312 = invoke class="VI" method="Abort VI"(reference=w519) -> (error out=w518:errorcluster)  [unwired: 2 in, 2 out]
        n313 = invoke class="VI" method="Abort VI"(error in=w518) -> ()  [unwired: 2 in, 3 out]
      }
      event User Event {
        n314 = event-data() -> ("IDs"=w528:cluster{"RPC field ID":u16, "Unique ID":u16}, "String"=w527:string)  [unwired: 1 in]
        n315 = Bundle("IDs"=w528, "String"=w527) -> (w526:T9)  [unwired: 1 in]
        n316 = call <vilib>:"Retrieve RPC Response.vi"("RPC Response"=w526) -> ("Output"=w523:string[][])  [unwired: 10 in]
        n317 = Build Array (concatenate)(w521, w523) -> (w522:string[][])
        n318 = local write "Command Params"(w522) -> ()
        n319 = local write "Cmd Status"("" ("Cmd Status")) -> ()
      }
      event "Vision": Value Change {
        # "Enable/Disable Compression slider.\nHW USB is hard-coded into the camera"
        n320 = event-data() -> ("NewVal"=w535:u16)  [unwired: 1 in]
        n321 = Equal?(x=w535, y=u32 2 ("milliseconds to wait")) -> (x = y?=w533:bool)
        n322 = Select(t=T24."Disabled and Grayed Out" ("Disabled"), s=w533, f=T24."Enabled" ("Disabled")) -> (s? t:f=w530:T24)
        n323 = property on="Compression" class="Slide (strict)"("DisabledEnum"=w530) -> ()  [unwired: 2 in, 2 out]
      }
      event "Tree": Double Click {
        n324 = event-data() -> ("PlatMods"=w540:T27, "Tag"=w539:string)  [unwired: 1 in]
        n325 = Unbundle(w540) -> ("Shift"=w538:bool)  [unwired: 4 out]
        n326 = Not(x=w538) -> (.not. x?=w537:bool)
        n327 = call <vilib>:"NT Update Persistence.vi"("Persistence"=w537, "Name"=w539) -> ()  [unwired: 9 in, 1 out]
      }
    }
  }
  n328 = Select(t=3.0, s=w17, f=w9) -> ()  [unwired: 1 out]
  n329 = call-poly <vilib>:"NT Read Value.vi"("Name"="ShifterGauche") -> ("Numeric"=w7:dbl)  [unwired: 9 in, 1 out]
  n330 = while {
    tunnel: w67 -> [w544]
    i -> [w547]
    stop <- FALSE stop-if-true
    n331 = Wait (ms)(milliseconds to wait=u32 100) -> ()  [unwired: 1 out]
    n332 = case shown="\"Playback\"" "Rec Mode" {
      tunnel: w547 -> [_ _ w562]
      tunnel: [u32 2829099 ("Base Color") u32 11141120 ("Target Color") w551] -> w543
      frame "Stop", Default {
        # "Reset the color, extra updates don't cost much"
      }
      frame "Record" {
      }
      frame "Playback" {
        # "Playback"
        n333 = Quotient & Remainder(x=w562, y=u32 50 ("milliseconds to wait")) -> (x-y*floor(x/y)=w558:u32)  [unwired: 1 out]
        n334 = Divide(x=w558, y=u32 50 ("milliseconds to wait")) -> (x/y=w555:dbl)
        n335 = Multiply(x=6.283185307179586, y=w555) -> (x*y=w560:dbl)
        n336 = Sine(x=w560) -> (sin(x)=w559:dbl)
        n337 = Absolute Value(x=w559) -> (abs(x)=w552:dbl)
        n338 = call "Interpolate RGB Color.vi"("Proportion"=w552, "Target Color"=u32 30976, "Base Color"=u32 2829099) -> ("Result Color"=w551:u32)  [unwired: 8 in]
      }
    }
    n339 = property class="Pane"(reference=w544, "PaneColor"=w543) -> ()  [unwired: 1 in, 2 out]
  }
  n340 = Greater?(x=w7, y=110.0) -> ()  [unwired: 1 out]
  n341 = Less?(x=w7, y=60.0) -> ()  [unwired: 1 out]
  n342 = call-poly <vilib>:"NT Read Value.vi"("Name"="ShifterDroit") -> ("Numeric"=w3:dbl)  [unwired: 9 in, 1 out]
  n343 = local write "Dashboard Tab"(T1."Drive" ("Dashboard Tab")) -> ()
  n344 = Greater?(x=w3, y=110.0) -> ()  [unwired: 1 out]
  n345 = Less?(x=w3, y=60.0) -> ()  [unwired: 1 out]
  n346 = property on="On/Off" class="Bool (strict)"("Visible"=w35) -> ()  [unwired: 2 in, 2 out]
  n347 = property on="Motor" class="Clust (strict)"("Visible"=w35) -> ()  [unwired: 2 in, 2 out]
  n348 = property on="Progress" class="Clust (strict)"("Visible"=w35) -> ()  [unwired: 2 in, 2 out]
  n349 = property on="Test Ring" class="Ring (strict)"("Visible"=w35) -> ()  [unwired: 2 in, 2 out]
  n350 = property on="Rev/Fwd" class="Clust (strict)"("Visible"=w35) -> ()  [unwired: 2 in, 2 out]
  n351 = property on="Camera Settings" class="Clust (strict)"("Visible"=w35) -> ()  [unwired: 2 in, 2 out]
  n352 = local write "DB Camera Config"(w35) -> ()
  n353 = while {
    tunnel: u16 1741 ("timeout ms (25000)") -> [w564]
    stop <- FALSE stop-if-true
    n354 = TCP Create Listener(10:w564) -> (0:w563:errorcluster, 3:w565:refnum<k5>)  [unwired: 4 in, 1 out]
    n355 = case shown="No Error" w563 {
      selector: w563 -> [w567 _]
      tunnel: w565 -> [w568 _]
      frame No Error {
        n356 = while {
          tunnel: w568 -> [w571]
          tunnel: w567 -> [w570]
          stop <- FALSE stop-if-true
          n357 = TCP Wait On Listener(8:w570, 11:w571) -> (0:w572:errorcluster, 4:w573:refnum<k5>)  [unwired: 2 in, 3 out]
          n358 = local write "TCP"(w573) -> ()
          n359 = case shown="No Error" w572 {
            frame No Error {
            }
            frame Error {
              n360 = Wait (ms)(milliseconds to wait=u32 1000) -> ()  [unwired: 1 out]
            }
          }
        }
      }
      frame Error {
        n361 = Wait (ms)(milliseconds to wait=u32 1000) -> ()  [unwired: 1 out]
      }
    }
  }
  n362 = local write "Command Params"(string[][] [] ("Command Params")) -> ()
  n363 = global write "WPI_DashboardLogging Global.vi" "Recording"(w61) -> ()
  n364 = local write "Rec Mode"(w61) -> ()
  n365 = local write "Command Selection"(u16 0 ("milliseconds to wait")) -> ()
